vi "PS and Spares Global.vi"() -> ()   [LabVIEW 2013]
panel:
  out "PS and Spares":fxp<+/-,28,17>[](array[numeric])
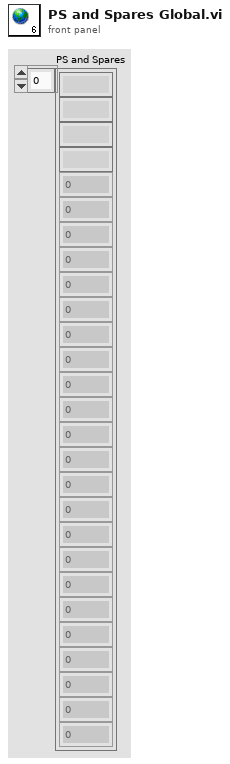
[diagram p1: front panel]
diagram:
